vi "datToWav.vi"() -> ()   [LabVIEW 2012]
panel:
  in  "dat File":path
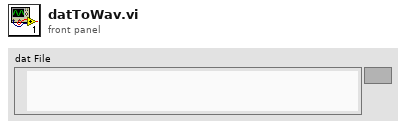
[diagram p1: front panel]
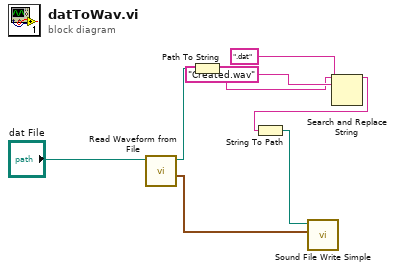
[diagram p0: block diagram]
diagram:
  n1 = call <vilib>:"Read Waveform from File.vi"("file path (dialog if empty)"="dat File") -> ("all waveforms in record"=w7:waveform(dbl)[], "new file path (Not A Path if cancelled)"=w4:path)  [unwired: 5 in, 2 out]
  n2 = Path To String(path=w4) -> (string=w3:string)
  n3 = Search and Replace String(input string=w3, search string="Created.wav", replace string=".dat" ("replace string (\"\")")) -> (result string=w2:string)  [unwired: 5 in, 3 out]
  n4 = String To Path(string=w2) -> (path=w1:path)
  n5 = call <vilib>:"Sound File Write Simple.vi"("data"=w7, "path"=w1) -> ()  [unwired: 8 in, 2 out]
